vi "sub-Get menu shortkey str.vi"(11 "menu desc":string) -> (2 "short key str":string, 3 "menu desc split":string)   [LabVIEW 2011]
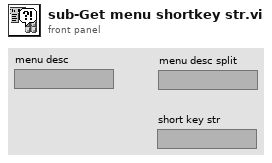
[diagram p1: front panel]
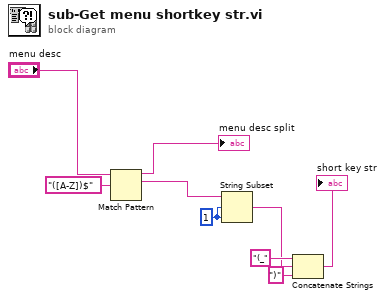
[diagram p0: block diagram]
diagram:
  w5 = 1 ("长度（剩余）")
  n1 = Match Pattern(string="menu desc", regular expression="([A-Z])$" ("正则表达式")) -> (before substring=→"menu desc split":string, match substring=w6:string)  [unwired: 1 in, 2 out]
  n2 = String Subset(string=w6, offset (0)=w5, length (rest)=w5) -> (substring=w3:string)
  n3 = Concatenate Strings("(_" ("字符串"), w3, ")" ("字符串")) -> (→"short key str":string)
